vi "PXDAC4800_SessionStreamEndXD48.vi"(0 "Handle":u32, 5 "Delete":bool) -> (4 "Status":i32)   [LabVIEW 2016]
uses:
  PXDAC4800.dll
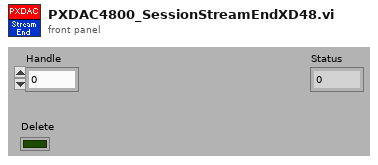
[diagram p1: front panel]
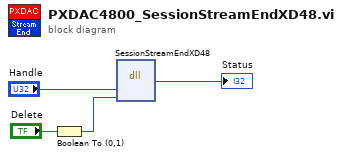
[diagram p0: block diagram]
diagram:
  n1 = Boolean To (0,1)(Boolean="Delete") -> (0, 1=w1:i16)
  n2 = dll-call lib="PXDAC4800.dll" fn="SessionStreamEndXD48"("Handle"="Handle", "Delete"=w1) -> (→"Status":i32)  [unwired: 5 in, 2 out]
